vi "Set Version Number.vi"(8 "error in (no error)":errorcluster, 10 "Version number":T1, 11 "SDIST in":refnum<class "NI_AB_API_SDIST.lvclass">) -> (0 "error out":errorcluster, 3 "SDIST out":refnum<class "NI_AB_API_SDIST.lvclass">)   [LabVIEW 2020, in "NI_AB_API_SDIST.lvclass"]
uses:
  <vilib>/AppBuilder/AB_API/SDIST/NI_AB_API_SDIST.lvclass
  <vilib>/AppBuilder/AB_API/common/AB_API Version Number.ctl
  <vilib>/AppBuilder/AB_API/Build/NI_AB_API_Build.lvclass
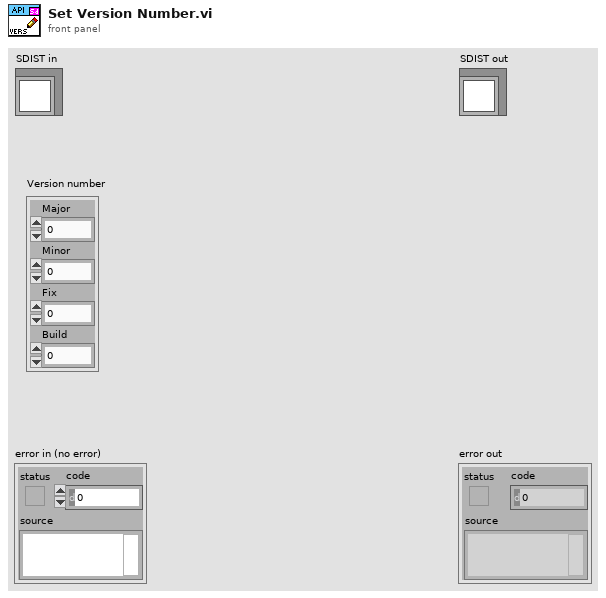
[diagram p1: front panel]
types:
  T1 = typedef "AB_API Version Number.ctl" = cluster{"Major":u16, "Minor":u16, "Fix":u16, "Build":u16}
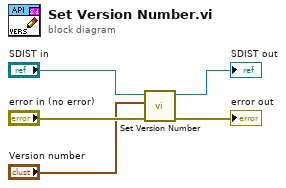
[diagram p0: block diagram]
diagram:
  n1 = call-parent "Set Version Number.vi"("error in (no error)"="error in (no error)", "Version number"="Version number", "NI_AB_API_Targetfile in"="SDIST in") -> ("error out"=→"error out":errorcluster, "NI_AB_API_Targetfile out"=→"SDIST out":refnum<class "NI_AB_API_SDIST.lvclass">)  [unwired: 7 in]
